vi "Create.vi"   [LabVIEW 2021, in "Field_RnD_Services_LIBSSH2_Toolkit.lvlib" / "Session.lvclass"]
doc: "Creates a new Session object that represents a libssh2lv shared library Session struct. This VI must be called, or executed, before using any other Session-related VIs. This VI allocates memory within the libssh2lv shared library that must be explicitly deallocated, or freed, at the end of the application using the <B>Destroy</B> VI to avoid memory leaks or running Out-of-Memory (OOM) on a resource contrained system.\n\nA Session object represents a connection to a remote SSH/SFTP server."
uses:
  220524-VNA RP FLAT.llb/Session.lvclass
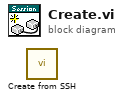
[diagram p0: block diagram]
diagram:
  n1 = call "Create from SSH.vi"() -> ()  [unwired: 10 in, 2 out]
